vi "RxChannel - Update Rx Channel Order.vi"(6 "Channel Names":string[](array[string]), 8 "error in (no error)":errorcluster, 11 "Node Ptr":T1 format="%.0x") -> (0 "error out":errorcluster, 3 "Node Ptr out":T1 format="%.0x")   [LabVIEW 2023, in "UDP-Custom-Device System Explorer.lvlib"]
uses:
  UDP-Custom-Device System Explorer.lvlib
  <vilib>/NI VeriStand/Custom Device API/Custom Device Item Ref.ctl
  <vilib>/NI VeriStand/Custom Device API/Custom Device API.lvlib
  Property Accessors/Rx Channel Section Accessors.lvlib
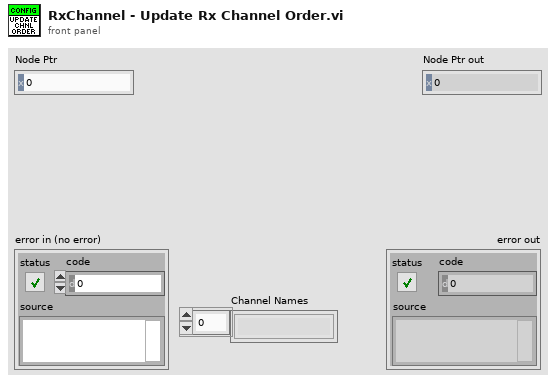
[diagram p1: front panel]
types:
  T1 = typedef "Custom Device API.lvlib/Custom Device Item Ref.ctl" = u64
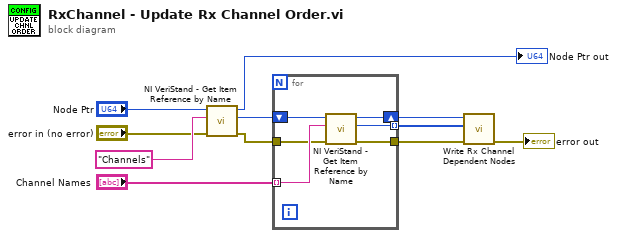
[diagram p0: block diagram]
diagram:
  n1 = call <vilib>:"NI VeriStand - Get Item Reference by Name.vi"("error in (no error)"="error in (no error)", "Item Name"="Channels" ("Section Name"), "Parent Ref in"="Node Ptr") -> ("error out"=w6:errorcluster, "Item Ref"=w8:T1, "Parent Ref out"=→"Node Ptr out":T1)  [unwired: 5 in, 1 out]
  n2 = for {
    tunnel: "Channel Names" -> [w16] mode=indexing
    tunnel: [w15] -> w3 mode=indexing
    tunnel: w6 -> [w13]
    shift-right: [w14] -> w4
    shift-left: w8 -> [w17]
    tunnel: [w12] -> w2
    n3 = call <vilib>:"NI VeriStand - Get Item Reference by Name.vi"("error in (no error)"=w13, "Item Name"=w16, "Parent Ref in"=w17) -> ("error out"=w12:errorcluster, "Item Ref"=w15:T1, "Parent Ref out"=w14:T1)  [unwired: 5 in, 1 out]
  }
  n4 = call "Write Rx Channel Dependent Nodes.vi"("error in (no error)"=w2, "Dependent Node Refs"=w3, "Node Ptr"=w4) -> ("error out"=→"error out":errorcluster)  [unwired: 7 in, 1 out]
